vi "GYRO_GET_RPY.vi"(9 "Invert_Yaw":bool, 10 "Invert_Pitch":bool, 11 "Invert_Roll":bool) -> (1 "Yaw_Deg":dbl, 2 "Pitch_Deg":dbl, 3 "Roll_Deg":dbl)   [LabVIEW 2023]
uses:
  SWERVE_DRIVE_GLOBALS.vi
  <vilib>/Rock Robotics/WPI/ThirdParty/Phoenix-LabVIEW/Pigeon IMU/CTRE_PigeonIMU_GetYPR.vi
  <vilib>/Rock Robotics/WPI/ThirdParty/Phoenix6/getters/GetPigeon2Yaw.vi
  <vilib>/Rock Robotics/WPI/ThirdParty/Phoenix6/getters/GetPigeon2Roll.vi
  <vilib>/Rock Robotics/WPI/ThirdParty/Phoenix6/getters/GetPigeon2Pitch.vi
  <vilib>/Rock Robotics/WPI/ThirdParty/JAS_Junk/TrajLib/Trajectory_Library.lvlib
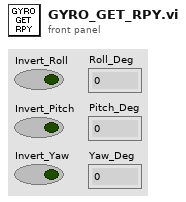
[diagram p1: front panel]
types:
  T1 = enum16{"Pigeon 2.0, P5", "Pigeon 2.0, P6", "NavX"}
  T2 = typedef "CTRE_PigeonIMU_DeviceRef.ctl" = cluster{"DeviceStatus":errorcluster, "Device Number":u8, "Type":T3, "Device ID":u32, "Handle":u64, "UsageFrame":u32, "Library Path":path}
  T3 = typedef "CTRE_PigeonIMU_ConnectionType.ctl" = u32
  T4 = typedef "DeviceReference.ctl" = cluster{"CANbus Name":string, "Device Encoding":u32, "Device Name":string}
  T5 = cluster{"Value":dbl, "System Timestamp":dbl, "CANivore Timestamp":dbl, "ECU Timestamp":dbl}
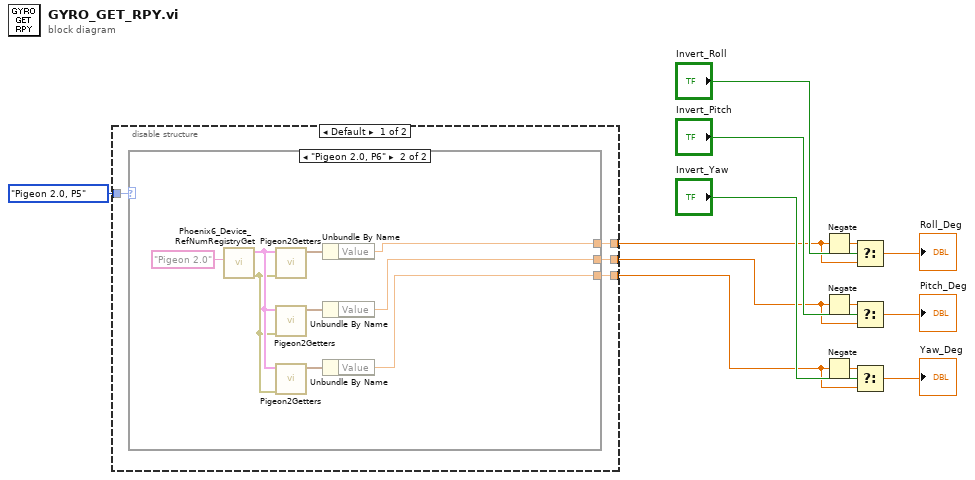
[diagram p0: block diagram]
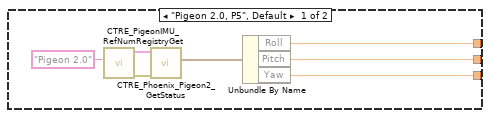
[diagram p2: hidden frame]
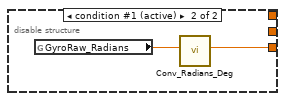
[diagram p3: hidden frame]
diagram:
  n1 = disable-structure shown="Default" {
    disable-tunnel: [w17 _] -> w6
    disable-tunnel: [w16 _] -> w5
    disable-tunnel: [w15 w34] -> w3
    disable-tunnel: T1."Pigeon 2.0, P5" ("MC type Drv") -> [w14 _]
    frame condition #0 {
      n2 = case shown="\"Pigeon 2.0, P6\"" w14 {
        tunnel: [w20 w27] -> w17
        tunnel: [w19 w26] -> w16
        tunnel: [w18 w25] -> w15
        frame "Pigeon 2.0, P5", Default {
          n3 = call <vilib>:"CTRE_PigeonIMU_RefNumRegistryGet.vi"("refnum name"="Pigeon 2.0") -> ("error out"=w24:errorcluster, "PigeonIMUDevRef"=w23:T2)  [unwired: 9 in]
          n4 = call-poly <vilib>:"CTRE_Phoenix_Pigeon2_GetStatus.vi"("error in (no error)"=w24, "PigeonIMUDevRef"=w23) -> ("Yaw Pitch Roll"=w22:cluster{"Yaw":dbl, "Pitch":dbl, "Roll":dbl})  [unwired: 7 in, 2 out]
          n5 = Unbundle By Name(w22) -> ("Roll"=w20:dbl, "Pitch"=w19:dbl, "Yaw"=w18:dbl)
        }
        frame "Pigeon 2.0, P6" {
          n6 = call <vilib>:"Phoenix6_Device_RefNumRegistryGet.vi"("refnum name"="Pigeon 2.0") -> ("error out"=w28:errorcluster, "data"=w29:T4)  [unwired: 9 in]
          n7 = call-poly <vilib>:"Pigeon2Getters.vi"("error in"=w28, "DeviceReference"=w29) -> ("Output"=w32:T5)  [unwired: 8 in, 1 out]
          n8 = call-poly <vilib>:"Pigeon2Getters.vi"("error in"=w28, "DeviceReference"=w29) -> ("Output"=w31:T5)  [unwired: 8 in, 1 out]
          n9 = call-poly <vilib>:"Pigeon2Getters.vi"("error in"=w28, "DeviceReference"=w29) -> ("Output"=w30:T5)  [unwired: 8 in, 1 out]
          n10 = Unbundle By Name(w32) -> ("Value"=w27:dbl)
          n11 = Unbundle By Name(w31) -> ("Value"=w26:dbl)
          n12 = Unbundle By Name(w30) -> ("Value"=w25:dbl)
        }
      }
    }
    frame condition #1 (active) {
      n13 = global read "SWERVE_DRIVE_GLOBALS.vi" "GyroRaw_Radians"() -> (w35:dbl)
      n14 = call <vilib>:"Conv_Radians_Deg.vi"("Radians"=w35) -> ("Degrees"=w34:dbl)  [unwired: 10 in]
    }
  }
  n15 = Negate(x=w6) -> (-x=w13:dbl)
  n16 = Negate(x=w5) -> (-x=w11:dbl)
  n17 = Negate(x=w3) -> (-x=w10:dbl)
  n18 = Select(t=w13, s="Invert_Roll", f=w6) -> (s? t:f=→"Roll_Deg":dbl)
  n19 = Select(t=w11, s="Invert_Pitch", f=w5) -> (s? t:f=→"Pitch_Deg":dbl)
  n20 = Select(t=w10, s="Invert_Yaw", f=w3) -> (s? t:f=→"Yaw_Deg":dbl)
